vi "RELAY_VI.vi"() -> ()   [LabVIEW 2022 SP3]
uses:
  <extravilib>/ChannelInstances/Tag-dbl/Read With Abort.vi
  <extravilib>/ChannelInstances/Stream-a[.](dbl)/Read With Abort.vi
  <extravilib>/ChannelInstances/Stream-a[.](dbl)/EndpointRead.vi
  <extravilib>/ChannelInstances/Stream-a[.](dbl)/Instantiate.vi
  <extravilib>/ChannelInstances/Stream-a[.](dbl)/)Channel.vi
  <resource>/ChannelSupport/_ChannelSupport/WaitIfNeeded.vi
  <extravilib>/ChannelInstances/Tag-dbl/Instantiate.vi
  <extravilib>/ChannelInstances/Tag-dbl/EndpointRead.vi
  <extravilib>/ChannelInstances/Tag-a[.](dbl).lvlib
panel:
  out "TrykHoej":dbl[](array[numeric])
  out "TrykLav":dbl[](array[numeric])
  in  "stop 4":bool
  in  "stop 3":bool
  in  "Ventil":bool
  in  "Pumpe":bool
  in  "Motor":bool
  in  "Kompressor":bool
  in  "stop":bool
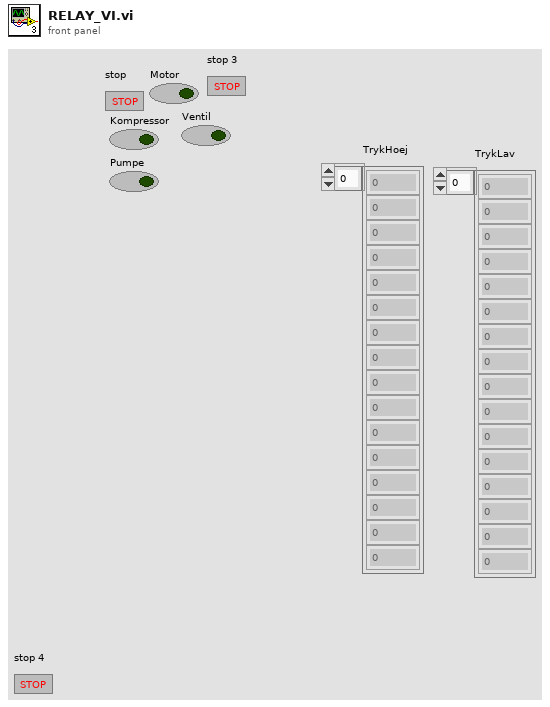
[diagram p1: front panel]
types:
  T1 = typedef "Tag-a[.](dbl).lvlib/))Channel.ctl" = refnum<queue>
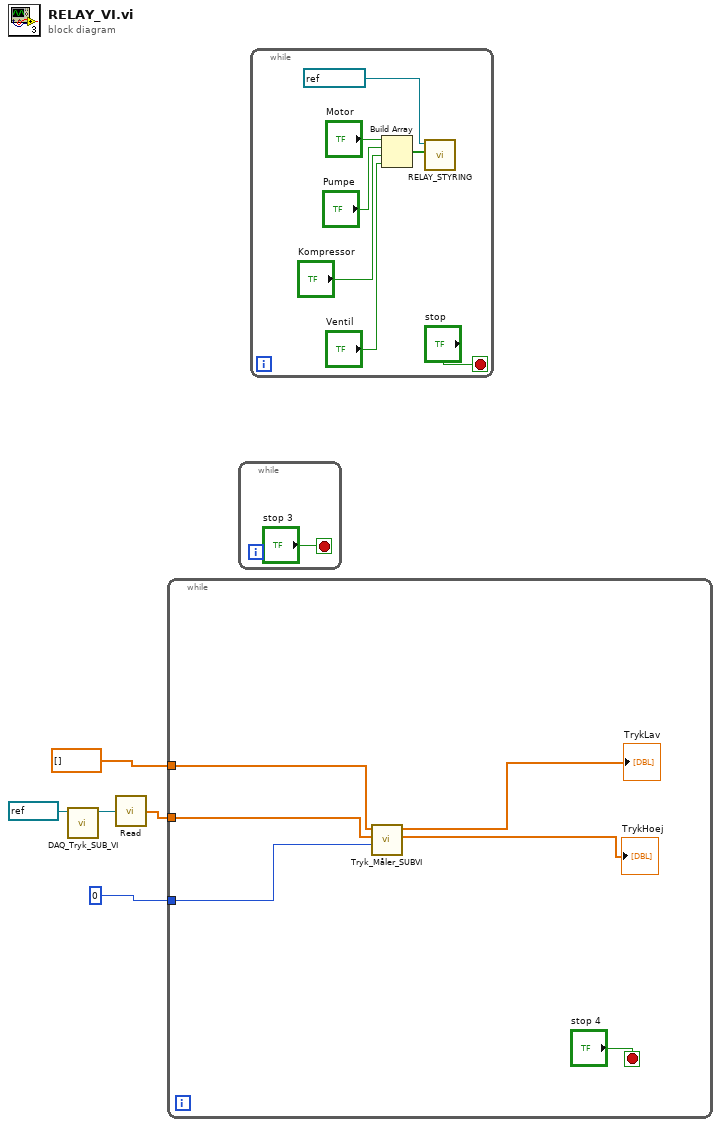
[diagram p0: block diagram]
diagram:
  n1 = call "DAQ_Tryk_SUB_VI.vi"("task in"=refnum<k21> "Tryk") -> ("channel"=w2:T1)  [unwired: 10 in]
  n2 = call <extravilib>:"Read.vi"("channel"=w2) -> ("element"=w1:dbl[])  [unwired: 1 in, 1 out]
  n3 = while {
    tunnel: 0 ("index") -> [w11]
    tunnel: dbl[] [] -> [w8]
    tunnel: w1 -> [w6]
    stop <- "stop 4" stop-if-true
    n4 = call "Tryk_Måler_SUBVI.vi"(9:w11, "element"=w6, "Array in"=w8) -> ("Tryk_Hoej"=→"TrykHoej":dbl[], "Tryk_Lav"=→"TrykLav":dbl[])  [unwired: 7 in]
  }
  n5 = while {
    stop <- "stop 3" stop-if-true
  }
  n6 = while {
    stop <- "stop" stop-if-true
    n7 = Build Array("Motor", "Pumpe", "Kompressor", "Ventil") -> (w13:bool[])
    n8 = call "RELAY_STYRING.vi"("data"=w13, "task/channels in"=refnum<k21> "RELAY") -> ()  [unwired: 10 in]
  }
